vi "TCP_Server(DAQ).vi"() -> ()   [LabVIEW 2019]
uses:
  9dddec59-2633-4920-86d0-fb84d7c00c5d.vi
  <vilib>/DAQmx/write.llb/DAQmx Write (Digital 1D Bool 1Chan 1Samp).vi
  <vilib>/DAQmx/miscellaneous.llb/DAQmx Fill In Error Info.vi
panel:
  out "ALTO":bool
  in  "Seguridad":bool=TRUE
  out "Recepción":string="\r\n"
  out "CORNETA":bool
  out "IZQUIERDA":bool
  out "DERECHA":bool
  out "CENTRO":bool
  out "ATRAS":bool
  out "ADELANTE":bool
  out "PUERTA":bool
  out "LUZ":bool
  out "Coincidencia":bool
  in  "stop":bool
  in  "listening port":u16=4900
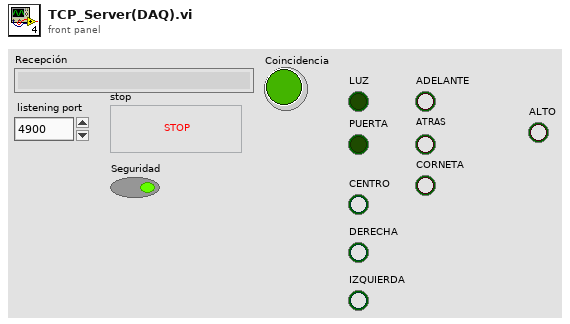
[diagram p1: front panel]
types:
  T1 = enum16{"Standard", "Buffered", "CRLF", "Immediate"}
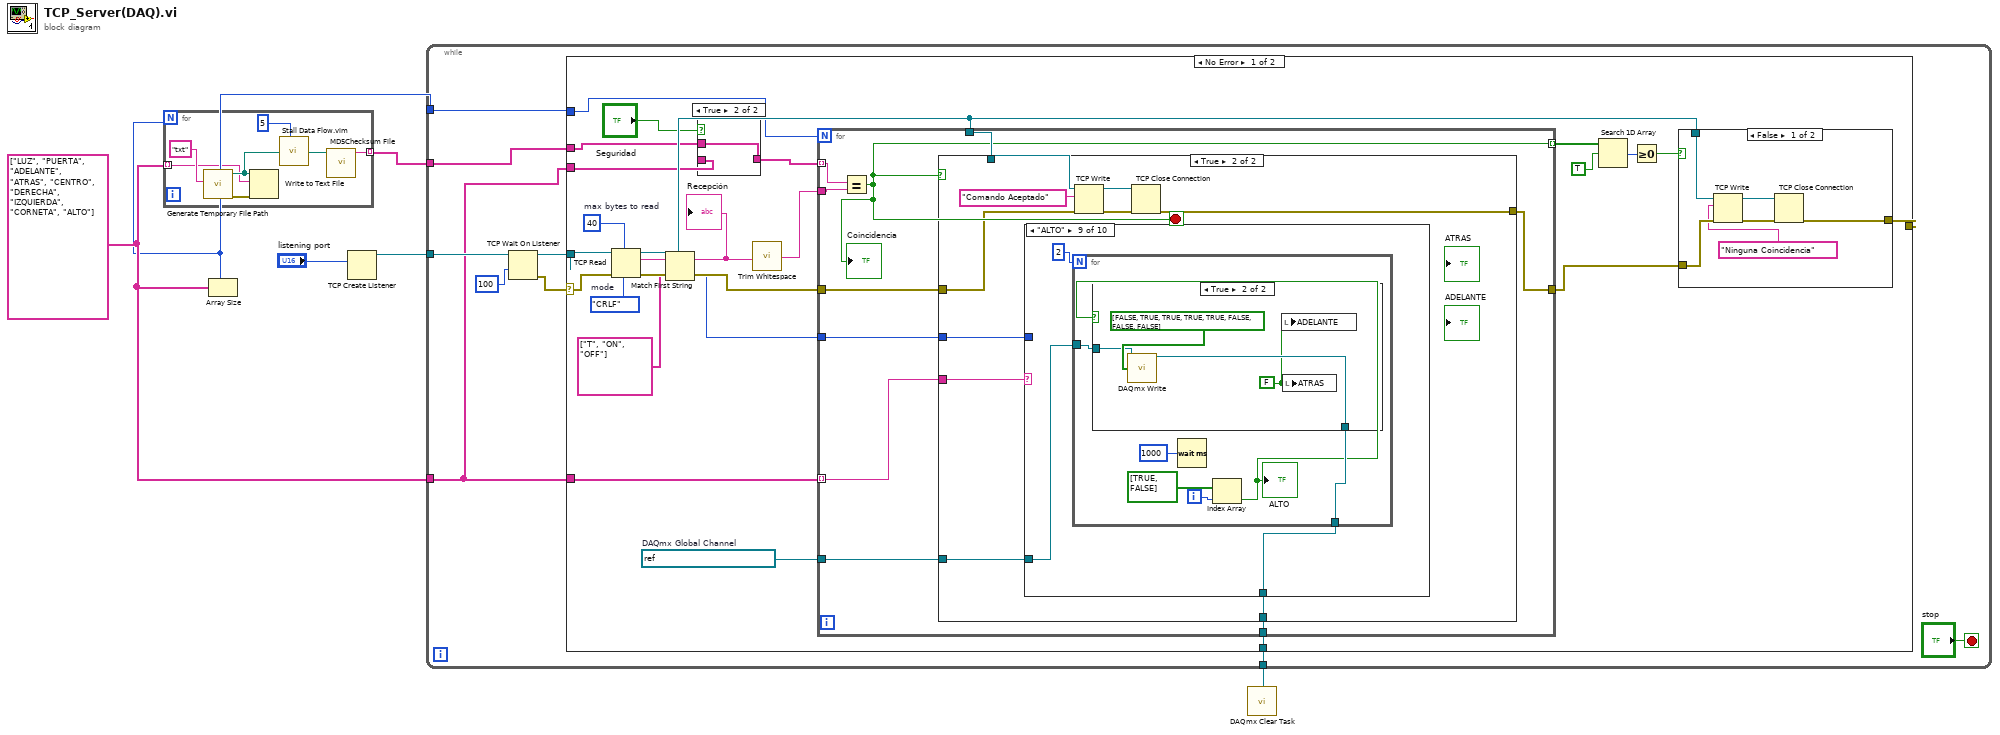
[diagram p0: block diagram]
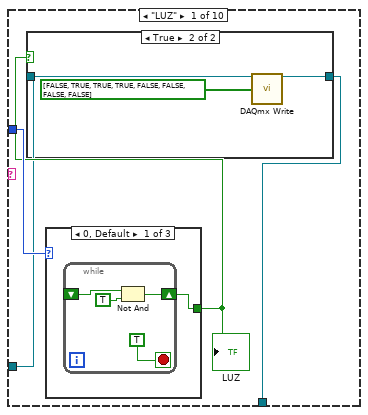
[diagram p5: hidden frame]
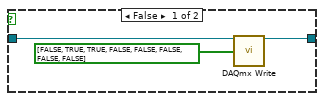
[diagram p6: hidden frame]
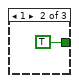
[diagram p7: hidden frame]
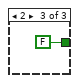
[diagram p8: hidden frame]
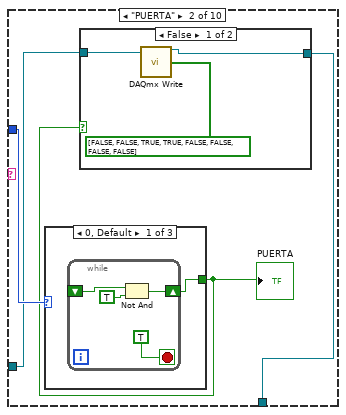
[diagram p9: hidden frame]
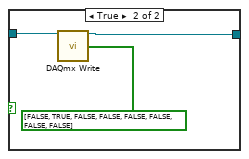
[diagram p10: hidden frame]
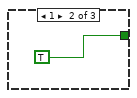
[diagram p11: hidden frame]
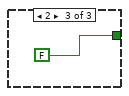
[diagram p12: hidden frame]
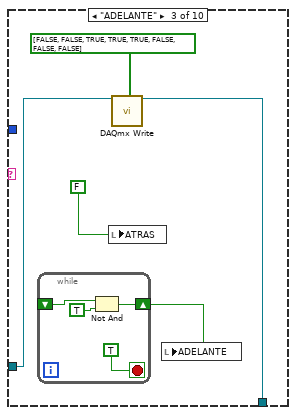
[diagram p13: hidden frame]
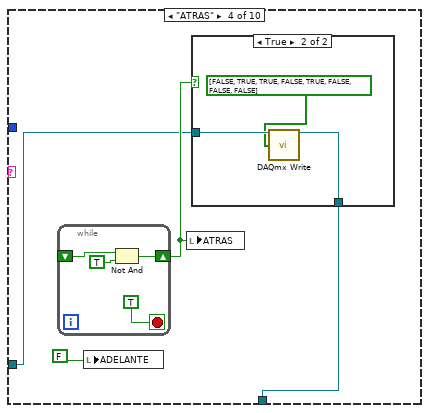
[diagram p14: hidden frame]
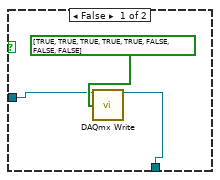
[diagram p15: hidden frame]
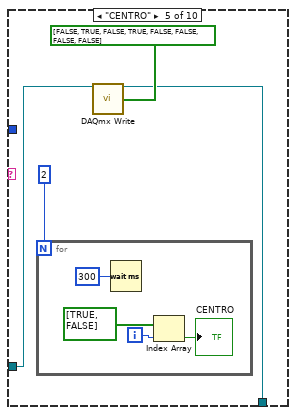
[diagram p16: hidden frame]
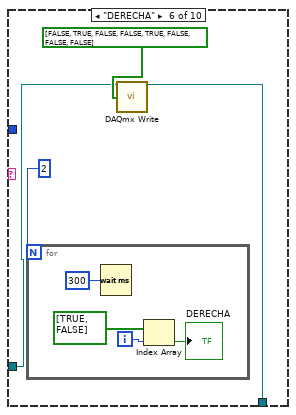
[diagram p17: hidden frame]
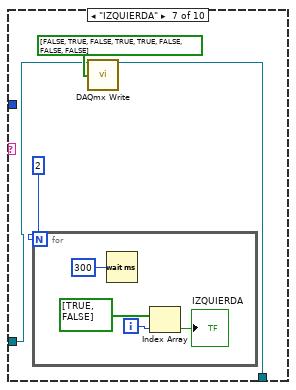
[diagram p18: hidden frame]
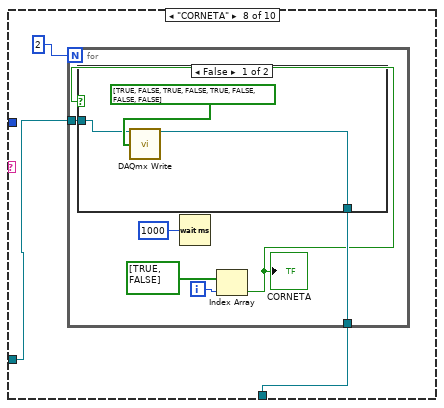
[diagram p19: hidden frame]
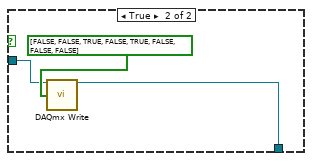
[diagram p20: hidden frame]
diagram:
  w2 = string[] ["LUZ", "PUERTA", "ADELANTE", "ATRAS", "CENTRO", "DERECHA", "IZQUIERDA", "CORNETA", "ALTO"]
  n1 = Array Size(array=w2) -> (size(s)=w1:i32)
  n2 = for {
    N: w1 -> [_]
    tunnel: w2 -> [w8] mode=indexing
    tunnel: [w7] -> w4 mode=indexing
    n3 = call <vilib>:"Generate Temporary File Path.vi"("Temporary File Extension (tmp)"="txt") -> ("error out"=w13:errorcluster, "Unique Temporary File Path"=w11:path)  [unwired: 9 in]
    n4 = Write to Text File(file (use dialog)=w11, text=w8, error in=w13) -> ()  [unwired: 1 in, 3 out]
    n5 = call "Stall Data Flow.vim"("value in"=w11, "milliseconds to wait"=u32 5) -> ("value out"=w12:path)  [unwired: 1 out]
    n6 = call <vilib>:"MD5Checksum File.vi"("Path"=w12) -> ("MD5 message-digest"=w7:string)  [unwired: 9 in, 1 out]
  }
  n7 = TCP Create Listener(10:"listening port") -> (3:w5:refnum<k5>)  [unwired: 4 in, 2 out]
  n8 = while {
    tunnel: w5 -> [w19]
    tunnel: w4 -> [w17]
    tunnel: w2 -> [w15]
    tunnel: [w16] -> w3
    tunnel: w1 -> [w14]
    stop <- "stop" stop-if-true
    n9 = TCP Wait On Listener(9:100 ("timeout ms (25000)"), 11:w19) -> (0:w22:errorcluster, 4:w20:refnum<k5>)  [unwired: 2 in, 3 out]
    n10 = case shown="No Error" w22 {
      selector: w22 -> [w45 w193]
      tunnel: [w34 w192] -> _
      tunnel: w20 -> [w44 _]
      tunnel: w17 -> [w26 _]
      tunnel: w15 -> [w41 _]
      tunnel: [w28 _] -> w16
      tunnel: w15 -> [w24 _]
      tunnel: w14 -> [w23 _]
      frame No Error {
        w29 = refnum<k21> "MyDigitalOutChannel"  # DAQmx Global Channel
        w47 = 40  # max bytes to read
        w46 = T1."CRLF"  # mode
        n11 = TCP Read(connection ID=w44, bytes to read=w47, error in (no error)=w45, 7:w46) -> (connection ID out=w36:refnum<k5>, data out=w32:string, error out=w42:errorcluster)  [unwired: 1 in]
        n12 = Match First String(2:string[] ["T", "ON", "OFF"] ("string array"), 3:w32) -> (0:w30:i32, 1:w31:string)
        "Recepción" <- w31
        n13 = case shown="True" "Seguridad" {
          tunnel: w26 -> [_ w49]
          tunnel: [w48 w49] -> w25
          tunnel: w24 -> [w48 _]
          frame False {
          }
          frame True {
          }
        }
        n14 = call <vilib>:"Trim Whitespace.vi"("string"=w31) -> ("trimmed string"=w43:string)  [unwired: 1 in]
        n15 = for {
          N: w23 -> [_]
          tunnel: w25 -> [w66] mode=indexing
          tunnel: w43 -> [w65]
          tunnel: w36 -> [w64]
          tunnel: w42 -> [w63]
          tunnel: [w61] -> w35
          tunnel: w41 -> [w60] mode=indexing
          tunnel: [w62] -> w38 mode=indexing
          tunnel: w30 -> [w59]
          tunnel: w29 -> [w58]
          tunnel: [w57] -> w28
          stop <- w62 stop-if-true
          n16 = Equal?(x=w65, y=w66) -> (x = y?=w62:bool)
          "Coincidencia" <- w62
          n17 = case shown="True" w62 {
            tunnel: w64 -> [_ w75]
            tunnel: w63 -> [w67 w74]
            tunnel: [w67 w73] -> w61
            tunnel: w60 -> [_ w72]
            tunnel: w59 -> [_ w71]
            tunnel: w58 -> [_ w70]
            tunnel: [_ w69] -> w57
            frame False {
            }
            frame True {
              n18 = case shown="\"ALTO\"" w72 {
                tunnel: w71 -> [w81 w98 _ _ _ _ _ _ _ _]
                tunnel: w70 -> [w79 w96 w113 w122 w136 w144 w152 w159 w176 w190]
                tunnel: [w78 w95 w112 w121 w135 w143 w151 w160 w175 w190] -> w69
                frame "LUZ" {
                  n19 = case shown="0, Default" w81 {
                    tunnel: [w88 TRUE FALSE] -> w80
                    frame 0, Default {
                      n20 = while {
                        shift-right: [w90] -> w88
                        shift-left: _ -> [w89]
                        stop <- TRUE stop-if-true
                        n21 = Not And(1:TRUE ("y"), 2:w89) -> (0:w90:bool)
                      }
                    }
                    frame 1 {
                    }
                    frame 2 {
                    }
                  }
                  "LUZ" <- w80
                  n22 = case shown="True" w80 {
                    tunnel: w79 -> [w83 w86]
                    tunnel: [w82 w85] -> w78
                    frame False {
                      n23 = call-poly <vilib>:"DAQmx Write.vi"("task/channels in"=w83, "data"=bool[] [FALSE, TRUE, TRUE, FALSE, FALSE, FALSE, FALSE, FALSE]) -> ("task out"=w82:refnum<k21>)  [unwired: 11 in, 2 out]
                    }
                    frame True {
                      n24 = call-poly <vilib>:"DAQmx Write.vi"("task/channels in"=w86, "data"=bool[] [FALSE, TRUE, TRUE, TRUE, FALSE, FALSE, FALSE, FALSE]) -> ("task out"=w85:refnum<k21>)  [unwired: 11 in, 2 out]
                    }
                  }
                }
                frame "PUERTA" {
                  n25 = case shown="0, Default" w98 {
                    tunnel: [w105 TRUE FALSE] -> w97
                    frame 0, Default {
                      n26 = while {
                        shift-right: [w107] -> w105
                        shift-left: _ -> [w106]
                        stop <- TRUE stop-if-true
                        n27 = Not And(1:TRUE ("y"), 2:w106) -> (0:w107:bool)
                      }
                    }
                    frame 1 {
                    }
                    frame 2 {
                    }
                  }
                  "PUERTA" <- w97
                  n28 = case shown="False" w97 {
                    tunnel: w96 -> [w100 w103]
                    tunnel: [w99 w102] -> w95
                    frame False {
                      n29 = call-poly <vilib>:"DAQmx Write.vi"("task/channels in"=w100, "data"=bool[] [FALSE, FALSE, TRUE, TRUE, FALSE, FALSE, FALSE, FALSE]) -> ("task out"=w99:refnum<k21>)  [unwired: 11 in, 2 out]
                    }
                    frame True {
                      n30 = call-poly <vilib>:"DAQmx Write.vi"("task/channels in"=w103, "data"=bool[] [FALSE, TRUE, FALSE, FALSE, FALSE, FALSE, FALSE, FALSE]) -> ("task out"=w102:refnum<k21>)  [unwired: 11 in, 2 out]
                    }
                  }
                }
                frame "ADELANTE" {
                  n31 = while {
                    shift-right: [w118] -> w116
                    shift-left: _ -> [w117]
                    stop <- TRUE stop-if-true
                    n32 = Not And(1:TRUE ("y"), 2:w117) -> (0:w118:bool)
                  }
                  n33 = local write "ATRAS"(FALSE) -> ()
                  n34 = call-poly <vilib>:"DAQmx Write.vi"("task/channels in"=w113, "data"=bool[] [FALSE, FALSE, TRUE, TRUE, TRUE, FALSE, FALSE, FALSE]) -> ("task out"=w112:refnum<k21>)  [unwired: 11 in, 2 out]
                  n35 = local write "ADELANTE"(w116) -> ()
                }
                frame "ATRAS" {
                  n36 = while {
                    shift-right: [w132] -> w123
                    shift-left: _ -> [w131]
                    stop <- TRUE stop-if-true
                    n37 = Not And(1:TRUE ("y"), 2:w131) -> (0:w132:bool)
                  }
                  n38 = local write "ADELANTE"(FALSE) -> ()
                  n39 = local write "ATRAS"(w123) -> ()
                  n40 = case shown="True" w123 {
                    tunnel: w122 -> [w125 w130]
                    tunnel: [w126 w128] -> w121
                    frame False {
                      n41 = call-poly <vilib>:"DAQmx Write.vi"("task/channels in"=w125, "data"=bool[] [TRUE, TRUE, TRUE, TRUE, TRUE, FALSE, FALSE, FALSE]) -> ("task out"=w126:refnum<k21>)  [unwired: 11 in, 2 out]
                    }
                    frame True {
                      n42 = call-poly <vilib>:"DAQmx Write.vi"("task/channels in"=w130, "data"=bool[] [FALSE, TRUE, TRUE, FALSE, TRUE, FALSE, FALSE, FALSE]) -> ("task out"=w128:refnum<k21>)  [unwired: 11 in, 2 out]
                    }
                  }
                }
                frame "CENTRO" {
                  n43 = for {
                    N: 2 -> [_]
                    i -> [w141]
                    n44 = Wait (ms)(milliseconds to wait=u32 300) -> ()  [unwired: 1 out]
                    n45 = Index Array(array=bool[] [TRUE, FALSE], index=w141) -> (element=→"CENTRO":bool)
                  }
                  n46 = call-poly <vilib>:"DAQmx Write.vi"("task/channels in"=w136, "data"=bool[] [FALSE, TRUE, FALSE, TRUE, FALSE, FALSE, FALSE, FALSE]) -> ("task out"=w135:refnum<k21>)  [unwired: 11 in, 2 out]
                }
                frame "DERECHA" {
                  n47 = for {
                    N: 2 -> [_]
                    i -> [w149]
                    n48 = Wait (ms)(milliseconds to wait=u32 300) -> ()  [unwired: 1 out]
                    n49 = Index Array(array=bool[] [TRUE, FALSE], index=w149) -> (element=→"DERECHA":bool)
                  }
                  n50 = call-poly <vilib>:"DAQmx Write.vi"("task/channels in"=w144, "data"=bool[] [FALSE, TRUE, FALSE, FALSE, TRUE, FALSE, FALSE, FALSE]) -> ("task out"=w143:refnum<k21>)  [unwired: 11 in, 2 out]
                }
                frame "IZQUIERDA" {
                  n51 = for {
                    N: 2 -> [_]
                    i -> [w157]
                    n52 = Wait (ms)(milliseconds to wait=u32 300) -> ()  [unwired: 1 out]
                    n53 = Index Array(array=bool[] [TRUE, FALSE], index=w157) -> (element=→"IZQUIERDA":bool)
                  }
                  n54 = call-poly <vilib>:"DAQmx Write.vi"("task/channels in"=w152, "data"=bool[] [FALSE, TRUE, FALSE, TRUE, TRUE, FALSE, FALSE, FALSE]) -> ("task out"=w151:refnum<k21>)  [unwired: 11 in, 2 out]
                }
                frame "CORNETA" {
                  n55 = for {
                    N: 2 -> [_]
                    tunnel: [w164] -> w160
                    tunnel: w159 -> [w163]
                    i -> [w166]
                    n56 = Wait (ms)(milliseconds to wait=u32 1000) -> ()  [unwired: 1 out]
                    n57 = Index Array(array=bool[] [TRUE, FALSE], index=w166) -> (element=w162:bool)
                    "CORNETA" <- w162
                    n58 = case shown="False" w162 {
                      tunnel: w163 -> [w168 w172]
                      tunnel: [w169 w171] -> w164
                      frame False {
                        n59 = call-poly <vilib>:"DAQmx Write.vi"("task/channels in"=w168, "data"=bool[] [TRUE, FALSE, TRUE, FALSE, TRUE, FALSE, FALSE, FALSE]) -> ("task out"=w169:refnum<k21>)  [unwired: 11 in, 2 out]
                      }
                      frame True {
                        n60 = call-poly <vilib>:"DAQmx Write.vi"("task/channels in"=w172, "data"=bool[] [FALSE, FALSE, TRUE, FALSE, TRUE, FALSE, FALSE, FALSE]) -> ("task out"=w171:refnum<k21>)  [unwired: 11 in, 2 out]
                      }
                    }
                  }
                }
                frame "ALTO" {
                  n61 = for {
                    N: 2 -> [_]
                    tunnel: [w179] -> w175
                    tunnel: w176 -> [w177]
                    i -> [w181]
                    n62 = Wait (ms)(milliseconds to wait=u32 1000) -> ()  [unwired: 1 out]
                    n63 = Index Array(array=bool[] [TRUE, FALSE], index=w181) -> (element=w178:bool)
                    "ALTO" <- w178
                    n64 = case shown="True" w178 {
                      tunnel: [w184 w188] -> w179
                      tunnel: w177 -> [w183 w187]
                      frame False {
                        n65 = call-poly <vilib>:"DAQmx Write.vi"("task/channels in"=w183, "data"=bool[] [TRUE, TRUE, TRUE, TRUE, TRUE, FALSE, FALSE, FALSE]) -> ("task out"=w184:refnum<k21>)  [unwired: 11 in, 2 out]
                      }
                      frame True {
                        w186 = FALSE ("ATRAS")
                        n66 = call-poly <vilib>:"DAQmx Write.vi"("task/channels in"=w187, "data"=bool[] [FALSE, TRUE, TRUE, TRUE, TRUE, FALSE, FALSE, FALSE]) -> ("task out"=w188:refnum<k21>)  [unwired: 11 in, 2 out]
                        n67 = local write "ADELANTE"(w186) -> ()
                        n68 = local write "ATRAS"(w186) -> ()
                      }
                    }
                  }
                }
                frame Default {
                }
              }
              n69 = TCP Write(connection ID=w75, data in="Comando Aceptado", error in (no error)=w74) -> (connection ID out=w77:refnum<k5>, error out=w76:errorcluster)  [unwired: 1 in, 1 out]
              n70 = TCP Close Connection(connection ID=w77, error in (no error)=w76) -> (error out=w73:errorcluster)  [unwired: 1 in, 1 out]
            }
          }
        }
        n71 = Search 1D Array(1D array=w38, element=TRUE) -> (index of element=w39:i32)  [unwired: 1 in]
        n72 = Greater Or Equal To 0?(x=w39) -> (x >= 0?=w37:bool)
        n73 = case shown="False" w37 {
          tunnel: w36 -> [w53 _]
          tunnel: w35 -> [w52 w56]
          tunnel: [w50 w56] -> w34
          frame False {
            n74 = TCP Write(connection ID=w53, data in="Ninguna Coincidencia", error in (no error)=w52) -> (connection ID out=w55:refnum<k5>, error out=w54:errorcluster)  [unwired: 1 in, 1 out]
            n75 = TCP Close Connection(connection ID=w55, error in (no error)=w54) -> (error out=w50:errorcluster)  [unwired: 1 in, 1 out]
          }
          frame True {
          }
        }
      }
      frame Error {
        n76 = call <vilib>:"Clear Errors.vi"("error in (no error)"=w193, "specific error code to clear (0: all)"=56) -> ("error out"=w192:errorcluster)  [unwired: 4 in, 1 out]
      }
    }
  }
  n77 = call <vilib>:"DAQmx Clear Task.vi"("task in"=w3) -> ()  [unwired: 14 in, 1 out]
